vi "Direction Indication.vi"(6 "Temperature":u16, 7 "Time Limit":u16, 9 "new element/subarray 2":T1, 10 "Speed":u16) -> (1 "new element/subarray 3":T1)   [LabVIEW 2014, in "Files Library.lvlib"]
uses:
  Files Library.lvlib
  CONTROL/Recipes Indicators.ctl
  Global/ClockWise Global.vi
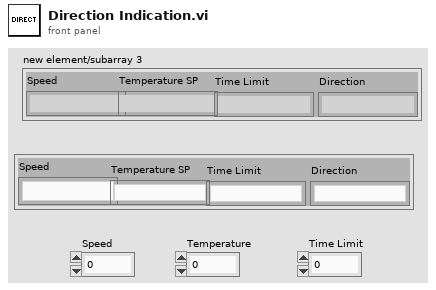
[diagram p1: front panel]
types:
  T1 = typedef "Recipes Indicators.ctl" = cluster{"Speed":string, "Temperature SP":string, "Time Limit":string, "Direction":string}
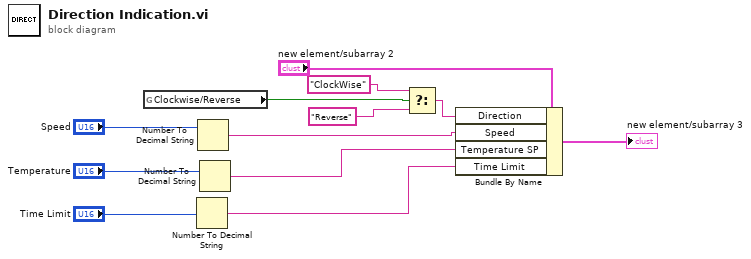
[diagram p0: block diagram]
diagram:
  n1 = global read "ClockWise Global.vi" "Clockwise/Reverse"() -> (w5:bool)
  n2 = Number To Decimal String(number="Time Limit") -> (decimal integer string=w7:string)  [unwired: 1 in]
  n3 = Number To Decimal String(number="Speed") -> (decimal integer string=w9:string)  [unwired: 1 in]
  n4 = Number To Decimal String(number="Temperature") -> (decimal integer string=w8:string)  [unwired: 1 in]
  n5 = Select(t="ClockWise", s=w5, f="Reverse") -> (s? t:f=w2:string)
  n6 = Bundle By Name(cluster="new element/subarray 2", "Direction"=w2, "Speed"=w9, "Temperature SP"=w8, "Time Limit"=w7) -> (→"new element/subarray 3":T1)
